vi "Avoid Obstacles.vi"(10 "Course Stage":dbl, 11 "Event":T1=enum."Start Button Pressed") -> (3 "Next State":u16)   [LabVIEW 2017]
uses:
  Event.ctl
  State.ctl
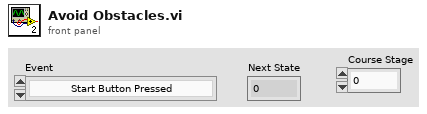
[diagram p1: front panel]
types:
  T1 = typedef "Event.ctl" = enum16{"None", "Zig Zag Finished", "Start Obstacle Avoidance", "Start Button Pressed", "Black & Yellow Tape Touched", "Black & Yellow Tape Passed", "Green Tape Crossed", "Red Tape Touched", "Rough Terrain Touched", "Black Tape Crossed", "Tape Edge Too Close", "Wall Too Close", "Rough Terrain Passed", "Ramp Passed", "Stop Button Pressed", "Recentered", "End Zone Wait Timed Out"}
  T2 = typedef "State.ctl" = enum16{"Wait", "Recenter", "Follow Wall", "Zig Zag", "Ramp", "Cross Rough Terrain", "Stagger Stop", "Obstacle Avoidance"}
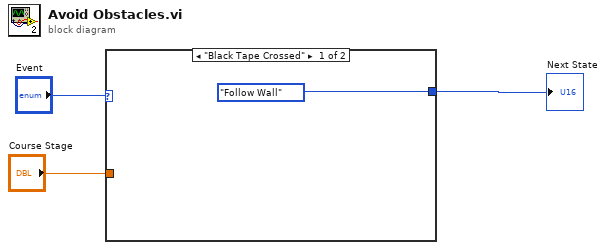
[diagram p0: block diagram]
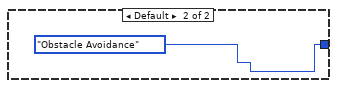
[diagram p2: hidden frame]
diagram:
  n1 = case shown="\"Black Tape Crossed\"" "Event" {
    tunnel: [State."Follow Wall" ("State") State."Obstacle Avoidance" ("State")] -> w2
    tunnel: "Course Stage" -> [_ _]
    frame "Black Tape Crossed" {
    }
    frame Default {
    }
  }
  "Next State" <- w2
